vi "Command Engine.vi"(8 "error in (no error)":errorcluster, 10 "Settings":T1 {"Compiled"."External Channels"."Channels" format="%.0x"; "Compiled"."External Channels"."Triggers" format="%.0x"}, 11 "Global Variables":T14) -> (0 "error out":errorcluster)   [LabVIEW 2018, in "Instrument Addon Engine.lvlib"]
uses:
  Instrument Addon Engine.lvlib
  <vilib>/NI/AMC/AMC.lvlib
  <vilib>/NI/NIVS Inline Async API/_VS Inline Async API/Process/Process.lvclass
  Types/Engine State Variables.ctl
  Addon Shared/Types/Linked Channel Cluster.ctl
  Addon Shared/Instrument Addon Shared.lvlib
  Addon Shared/Types/Command Parameters.ctl
  <vilib>/NI VeriStand/Custom Device API/Data Reference.ctl
  <vilib>/NI VeriStand/Custom Device API/Custom Device API.lvlib
  Types/Commands RT Configuration Cluster.ctl
  Addon Shared/Types/Response Wait Type.ctl
  Addon Shared/Types/Response Parameters.ctl
  Addon Shared/Types/Response RT Configuration Cluster.ctl
  Addon Shared/Types/Message Generation Type.ctl
  Addon Shared/Types/Message Parameters.ctl
  Addon Shared/Types/External Trigger Refs.ctl
  Addon Shared/Types/Compiled Settings.ctl
  Source/Addon/Support Libraries/Protections.lvlibp/Parent Protection/Protection.lvclass
  Source/Addon/Support Libraries/Protocols.lvlibp/Protocol Parent/Protocol Parent.lvclass
  <vilib>/NI/NIVS Inline Async API/_Data Access Engine/Access Type Classes/ReadWrite/ReadWrite.lvclass
  <vilib>/NI/NI VeriStand Addon Network Comm/Engine/VeriStand Comm.lvclass
  <vilib>/NI/NIVS Inline Async API/_Data Access Engine/Access Type Classes/Write/Write.lvclass
  <vilib>/NI/NIVS Inline Async API/_Data Access Engine/Data Access Engine/Types/Write.DVR.ctl
  <vilib>/NI/NIVS Inline Async API/_Data Access Engine/Data Access Engine/Data Access Engine.lvclass
  <vilib>/NI/NIVS Inline Async API/_Data Access Engine/Access Type Classes/Read/Read.lvclass
  <vilib>/NI/NIVS Inline Async API/_Data Access Engine/Data Access Engine/Types/Read.DVR.ctl
  <vilib>/NI/NIVS Inline Async API/_Data Access Engine/Data Access Engine/Types/ReadWrite.DVR.ctl
  Addon Shared/Types/Command Channel Index.ctl
  Addon Shared/Types/Command Channel Indeces.ctl
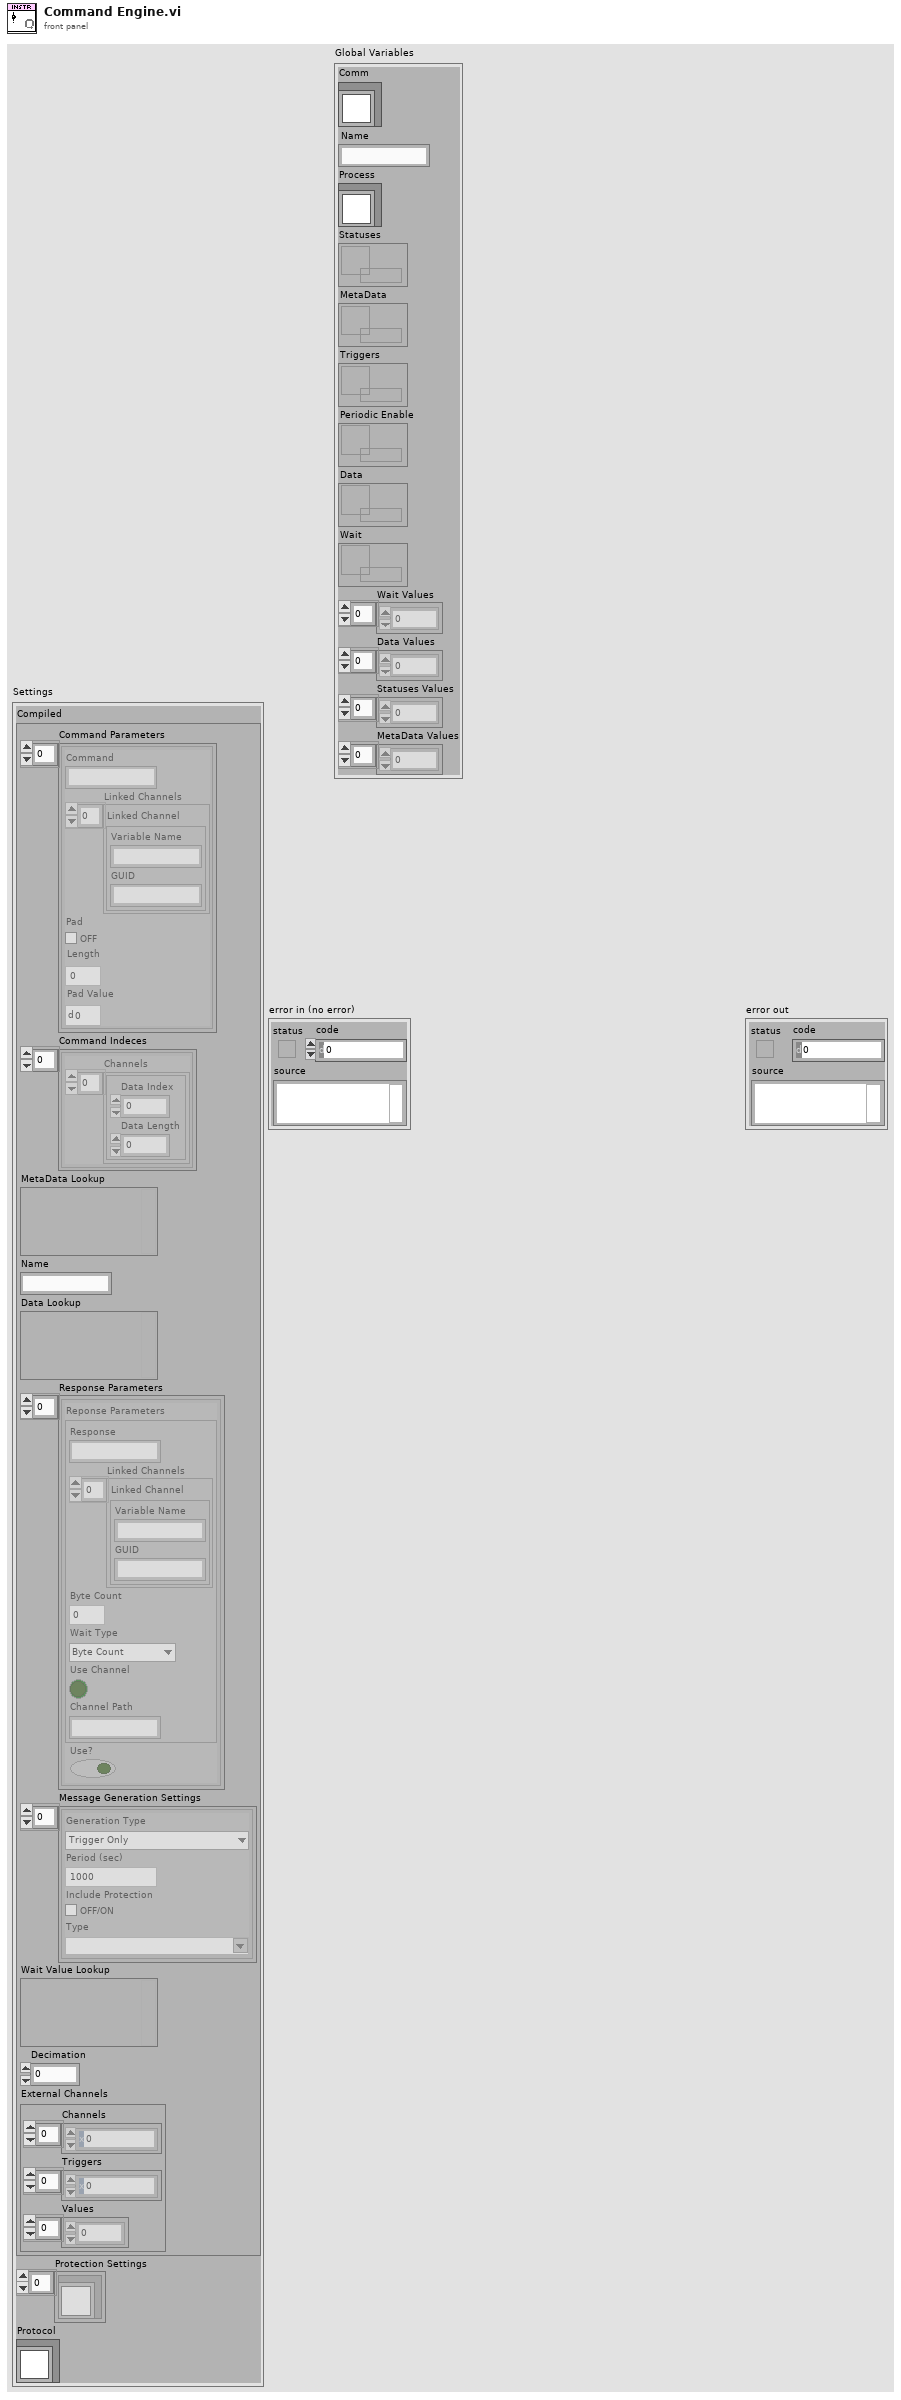
[diagram p1: front panel]
types:
  T1 = typedef "Instrument Addon Engine.lvlib/Commands RT Configuration Cluster.ctl" = cluster{"Compiled":T2, "Protection Settings":refnum<class "Protection.lvclass">[], "Protocol":refnum<class "Protocol Parent.lvclass">}
  T2 = typedef "Instrument Addon Shared.lvlib/Compiled Settings.ctl" = cluster{"Command Parameters":T3[], "Command Indeces":T5[], "MetaData Lookup":variant, "Name":string, "Data Lookup":variant, "Response Parameters":T7[], "Message Generation Settings":T10[], "Wait Value Lookup":variant, "Decimation":u32, "External Channels":T12}
  T3 = typedef "Instrument Addon Shared.lvlib/Command Parameters.ctl" = cluster{"Command":string, "Linked Channels":T4[], "Pad":bool, "Length":u32, "Pad Value":u8}
  T4 = typedef "Instrument Addon Shared.lvlib/Linked Channel Cluster.ctl" = cluster{"Variable Name":string, "GUID":string}
  T5 = typedef "Instrument Addon Shared.lvlib/Command Channel Indeces.ctl" = cluster{"Channels":T6[]}
  T6 = typedef "Instrument Addon Shared.lvlib/Command Channel Index.ctl" = cluster{"Data Index":i32, "Data Length":i32}
  T7 = typedef "Instrument Addon Shared.lvlib/Response RT Configuration Cluster.ctl" = cluster{"Reponse Parameters":T8, "Use?":bool}
  T8 = typedef "Instrument Addon Shared.lvlib/Response Parameters.ctl" = cluster{"Response":string, "Linked Channels":T4[], "Type Value":dbl, "Wait Type":T9, "Use Channel":bool, "Channel Path":string}
  T9 = typedef "Instrument Addon Shared.lvlib/Response Wait Type.ctl" = enum16{"Byte Count", "Wait sec"}
  T10 = typedef "Instrument Addon Shared.lvlib/Message Parameters.ctl" = cluster{"Generation Type":T11, "Period":dbl, "Include Protection":bool, "Type":string}
  T11 = typedef "Instrument Addon Shared.lvlib/Message Generation Type.ctl" = enum16{"Trigger Only", "Periodic & Trigger", "Value Change & Trigger"}
  T12 = typedef "Instrument Addon Shared.lvlib/External Trigger Refs.ctl" = cluster{"Channels":T13[], "Triggers":T13[], "Values":dbl[]}
  T13 = typedef "Custom Device API.lvlib/Data Reference.ctl" = i32
  T14 = typedef "Instrument Addon Engine.lvlib/Engine State Variables.ctl" = cluster{"Comm":refnum<class "VeriStand Comm.lvclass">, "Name":string, "Process":refnum<class "Process.lvclass">, "Statuses":T15, "MetaData":T16, "Triggers":T17, "Periodic Enable":T16, "Data":T15, "Wait":T16, "Wait Values":dbl[], "Data Values":dbl[], "Statuses Values":dbl[], "MetaData Values":dbl[]}
  T15 = typedef "Data Access Engine.lvlib/Data Access Engine.lvclass/Write.DVR.ctl" = refnum<data-value>
  T16 = typedef "Data Access Engine.lvlib/Data Access Engine.lvclass/Read.DVR.ctl" = refnum<data-value>
  T17 = typedef "Data Access Engine.lvlib/Data Access Engine.lvclass/ReadWrite.DVR.ctl" = refnum<data-value>
  T18 = typedef "Instrument Addon Engine.lvlib/command engine global variables.ctl" = cluster{"Time":u32[], "Triggers":bool[], "Rsp Queue":T19, "# of Messages":i32, "Rsp Attributes":T20}
  T19 = typedef "AMC.lvlib/Message Queue.ctl" = refnum<queue>
  T20 = typedef "Tools_KeyedArray.lvlib/KeyedArray.ctl" = cluster{"keys":string[], "values":string[]}
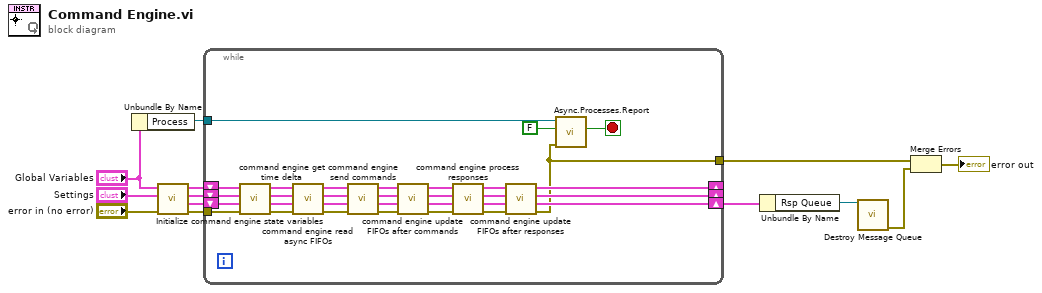
[diagram p0: block diagram]
diagram:
  n1 = Unbundle By Name("Global Variables") -> ("Process"=w13:refnum<class "Process.lvclass">)
  n2 = call "Initialize command engine state variables.vi"("error in (no error)"="error in (no error)", "Settings"="Settings", "Global Variables"="Global Variables") -> ("error out"=w10:errorcluster, "State Variables out"=w6:T18, "Settings out"=w7:T1, "Global Variables out"=w8:T14)  [unwired: 5 in]
  n3 = while {
    tunnel: w10 -> [w41]
    tunnel: [w14] -> w3
    tunnel: w13 -> [w42]
    shift-right: [w23] -> _
    shift-left: w8 -> [w18]
    shift-right: [w22] -> _
    shift-left: w7 -> [w19]
    shift-right: [w21] -> w5
    shift-left: w6 -> [w20]
    stop <- w44 stop-if-true
    n4 = call "command engine get time delta.vi"("error in (no error)"=w41, "State Variables in"=w20, "Settings"=w19, "Global Variables"=w18) -> ("error out"=w40:errorcluster, "State Variables out"=w16:T18, "Settings out"=w17:T1, "Global Variables out"=w15:T14)  [unwired: 4 in]
    n5 = call "command engine read async FIFOs.vi"("error in (no error)"=w40, "State Variables"=w16, "Settings"=w17, "Global Variables"=w15) -> ("error out"=w36:errorcluster, "State Variables out"=w38:T18, "Settings out"=w37:T1, "Global Variables out"=w39:T14)  [unwired: 4 in]
    n6 = call "command engine send commands.vi"("error in (no error)"=w36, "State Variables"=w38, "Settings"=w37, "Global Variables"=w39) -> ("error out"=w33:errorcluster, "State Variables out"=w34:T18, "Settings out"=w35:T1, "Global Variables out"=w32:T14)  [unwired: 4 in]
    n7 = call "command engine update FIFOs after commands.vi"("error out"=w33, "State Variables in"=w34, "Settings in"=w35, "Global Variables"=w32) -> ("error out"=w31:errorcluster, "State Variables out"=w30:T18, "Settings out"=w29:T1, "Global Variables out"=w28:T14)  [unwired: 4 in]
    n8 = call "command engine process responses.vi"("error out"=w31, "State Variables"=w30, "Settings"=w29, "Global Variables"=w28) -> ("error out"=w24:errorcluster, "State Variables out"=w25:T18, "Settings out"=w27:T1, "Global Variables out"=w26:T14)  [unwired: 4 in]
    n9 = call "command engine update FIFOs after responses.vi"("error out"=w24, "State Variables in"=w25, "Settings in"=w27, "Global Variables in"=w26) -> ("error out"=w14:errorcluster, "State Variables out"=w21:T18, "Settings out"=w22:T1, "Global Variables out"=w23:T14)  [unwired: 4 in]
    n10 = call <vilib>:"Async.Processes.Report.vi"("Error"=w14, "Stop Async on Error?"=FALSE ("Stop on Error?"), "Process in"=w42) -> ("Stop"=w44:bool)  [unwired: 7 in, 1 out]
  }
  n11 = Unbundle By Name(w5) -> ("Rsp Queue"=w4:T19)
  n12 = call <vilib>:"Destroy Message Queue.vi"("message queue in"=w4) -> ("error out"=w2:errorcluster)  [unwired: 12 in, 2 out]
  n13 = Merge Errors(w3, w2) -> (→"error out":errorcluster)
